vi "Cliente.vi"() -> ()   [LabVIEW 2024]
panel:
  out "*(type *) &x":dbl
  in  "stop":bool
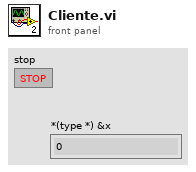
[diagram p1: front panel]
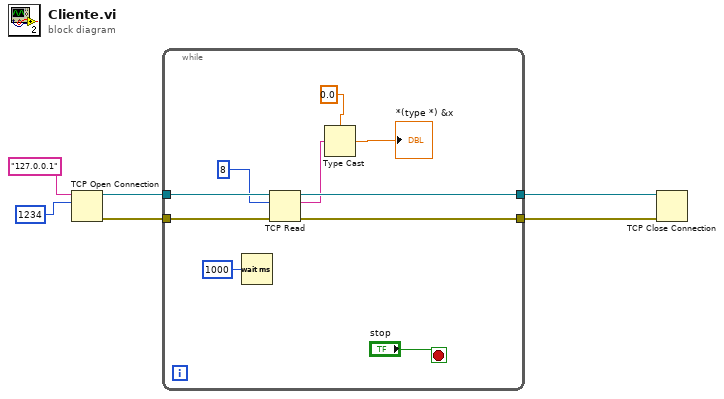
[diagram p0: block diagram]
diagram:
  n1 = TCP Open Connection(address="127.0.0.1", remote port or service name=u16 1234) -> (connection ID=w4:refnum<k5>, error out=w3:errorcluster)  [unwired: 3 in]
  n2 = while {
    tunnel: w4 -> [w16]
    tunnel: w3 -> [w15]
    tunnel: [w14] -> w2
    tunnel: [w13] -> w1
    stop <- "stop" stop-if-true
    n3 = Wait (ms)(milliseconds to wait=u32 1000) -> ()  [unwired: 1 out]
    n4 = TCP Read(connection ID=w16, bytes to read=8, error in (no error)=w15) -> (connection ID out=w14:refnum<k5>, data out=w7:string, error out=w13:errorcluster)  [unwired: 2 in]
    n5 = Type Cast(type=0.0, x=w7) -> (*(type *) &x=→"*(type *) &x":dbl)
  }
  n6 = TCP Close Connection(connection ID=w2, error in (no error)=w1) -> ()  [unwired: 1 in, 2 out]
